vi "Report build (SubVI).vi"(0 "Full/Fails":string(combo)="Full", 1 "Operator":string, 2 "Original ATR Ref":refnum<vi>, 3 "GeneralResult-Pass(T)Fail(F)":bool, 4 "Header Array":string[][](array[string]), 5 "error in (no error)":errorcluster, 6 "report file path":path, 8 "PN":string, 14 "SN":string) -> (19 "error out":errorcluster)   [LabVIEW 2017]
uses:
  <vilib>/Utility/miscctls.llb/LVRowAndColumnUnsignedTypeDef.ctl
  <vilib>/Utility/NIReport.llb/HTML Report Image Alignment.ctl
  <vilib>/Utility/NIReport.llb/Append Image to Report (path wrap).vi
  <vilib>/Utility/NIReport.llb/Append Report Text (str wrap).vi
  <vilib>/Utility/NIReport.llb/Append Text Table to Report (wrap).vi
  <vilib>/Utility/NIReport.llb/NI_report.lvclass
  <vilib>/Utility/NIReport.llb/Word/NI_Word.lvclass
  <vilib>/addons/_office/NI_ReportGenerationToolkit.lvlib
  <vilib>/Utility/NIReport.llb/NI_ReportGenerationCore.lvlib
panel:
  in  "ATR":string[][](table)=[["Comm. & Motor Test", "", "", "", "", "N/A", " ", "", "", "", "", " "], ["RS232 Communication", "", "-", "-", "N/A", "N/A", " ", "", "", "", "", ""], ["Version", "", "-", "-", "N/A", "N/A", "", "", "", "", "", ""], ["Motor Speed", "1000", "-", "-", "N/A", "N/A", "", "", "", "", "", ""], ["Motor Dir.", "1000", "-", "-", "N/A", "N/A", "", "", "", "", "", ""], ["", "", "", "", " ", " ", "", "", "", "", "", ""], ["Motor Thermistor Test", "", "", "", " ", "N/A", "", "", "", "", "", ""], ["Thermistor Disable", "0", "+/-100", "rpm", "N/A", "N/A", "", "", "", "", "", ""], ["Thermistor Enable", "1000", "+/-100", "rpm", "N/A", "N/A", "", "", "", "", "", ""], ["", "", "", "", "", "", "", "", "", "", "", ""], ["Motor Run Test", "", "", "", "", "", "", "", "", "", "", ""], ["Motor Temper. befor Run", "30", "+/-15", "C", "N/A", "N/A", "", "", "", "", "", ""], ["Motor Current after 1 min", "40", "+/-3", "A", "N/A", "N/A", "", "", "", "", "", ""], ["Motor Temper. after 20 min", "45", "+/-15", "C", "N/A", "N/A", "", "", "", "", "", ""], ["Motor Current after 20 min", "40", "+/-3", "A", "N/A", "N/A", "", "", "", "", "", ""], ["", "", "", "", "", "", "", "", "", "", "", ""], ["Visual Inspection Tests", "", "", "", "", "N/A", "", "", "", "", "", ""], ["", "", "", "", "", "", "", "", "", "", "", ""], ["Conductivity Test", "", "", "", "", "N/A", "", "", "", "", "", ""], ["J1 to Chasis", "< 2m", "-", "ohms", "N/A", "N/A", "", "", "", "", "", ""], ["", "", "", "", "", "", "", "", "", "", "", ""], ["Insulation Resistance Test", "", "", "", "", "N/A", "", "", "", "", "", ""], ["J1B", "> 500k", "-", "ohms", "N/A", "N/A", "", "", "", "", "", ""], ["J1E", "> 500k", "-", "ohms", "N/A", "N/A", "", "", "", "", "", ""], ["", "", "", "", "", "", "", "", "", "", "", ""], ["Blower Calibration", "", "", "", "", "N/A", "", "", "", "", "", ""], ["Motor Speed", "8000", "+/-100", "rpm", "N/A", "N/A", "", "", "", "", "", ""], ["Driver Current", "40", "+/-3", "A", "N/A", "N/A", "", "", "", "", "", ""], ["", "", "", "", "", "", "", "", "", "", "", ""], ["Leak Test", "", "", "", "", "N/A", "", "", "", "", "", ""], ["Leak Test", "5", "+/-0.2", "psig", "N/A", "N/A", "", "", "", "", "", ""], ["", "", "", "", "", "", "", "", "", "", "", ""], ["Set Production Parameters", "", "", "", "", "", "", "", "", "", "", ""], ["Unit Serial Number", "#6", "-", "-", "N/A", "N/A", "", "", "", "", "", ""], ["Unit Part Number", "#7", "-", "-", "RD00000", "N/A", "", "", "", "", "", ""]]
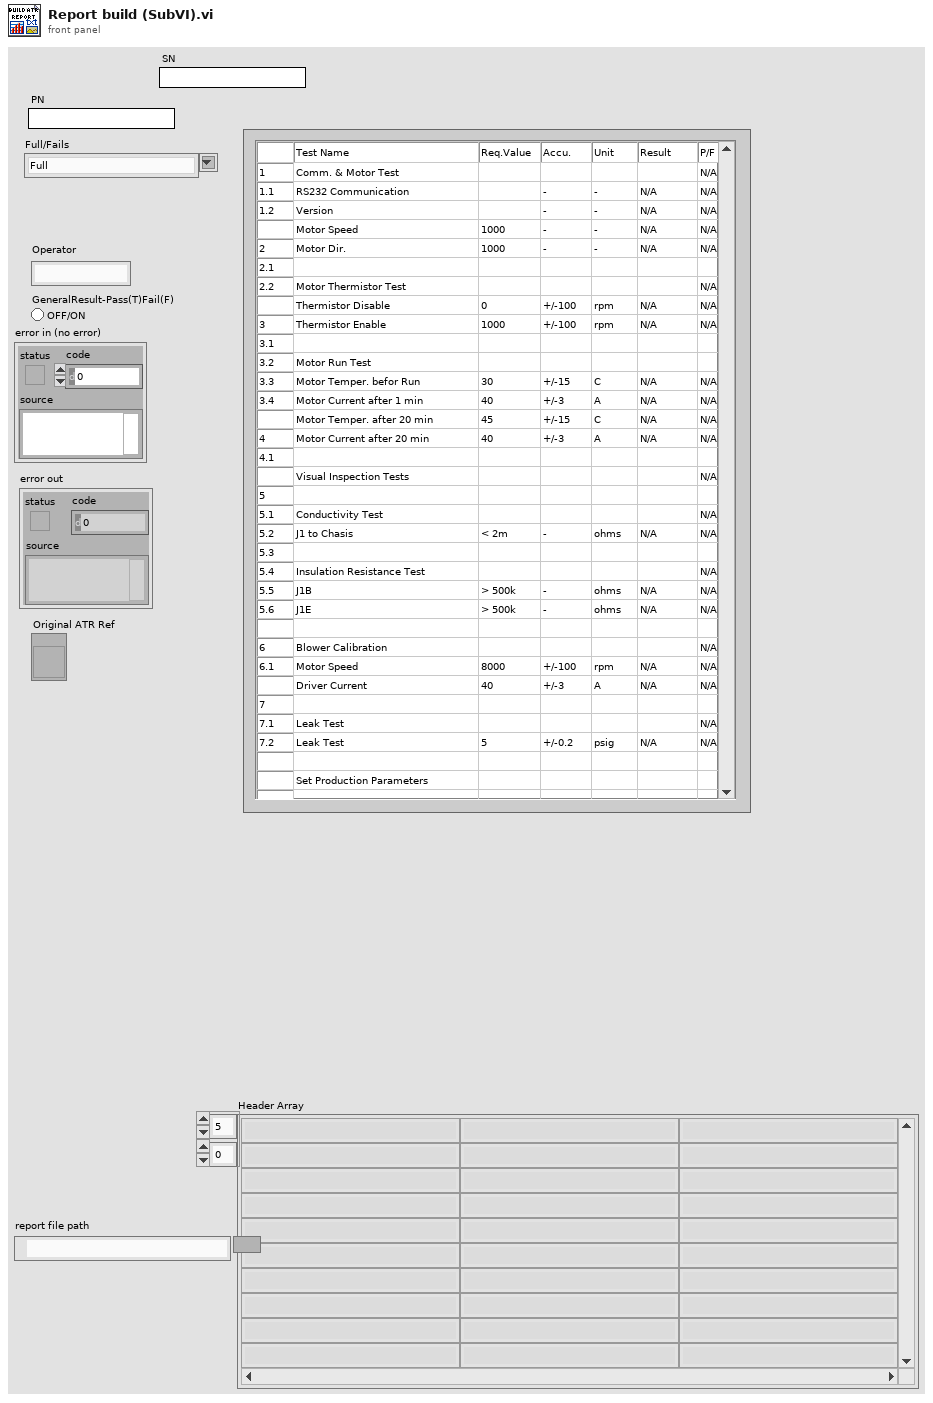
[diagram p1: front panel]
types:
  T1 = cluster{"top":dbl, "left":dbl, "right":dbl, "bottom":dbl}
  T2 = cluster{"alignment":enum16{"Left", "Centered", "Right", "Justify"}, "left":dbl, "right":dbl, "special":enum16{"(none)", "First line", "Hanging"}, "by":dbl, "before":dbl, "after":dbl, "line spacing":enum16{"Single", "1,5 lines", "Double", "At least", "Exactly", "Multiple"}, "at":dbl}
  T3 = enum16{"maximized", "minimized", "normal", "no change"}
  T4 = enum16{"Standard Report", "HTML", "Word", "Excel"}
  T5 = typedef "LVRowAndColumnUnsignedTypeDef.ctl" = cluster{"Row":u32, "Column":u32}
  T6 = typedef "LVFontTypeDef.ctl" = cluster{"Font Name":string, "Size":u16, "Bold":bool, "Italic":bool, "Underline":bool, "Strikeout":bool, "Color":u32}
  T7 = typedef "NI_ReportGenerationCore.lvlib/HTML Report Image Alignment.ctl" = enum16{"(default)", "LEFT", "RIGHT", "TOP", "TEXTTOP", "MIDDLE", "ABSMIDDLE", "BASELINE", "BOTTOM", "ABSBOTTOM"}
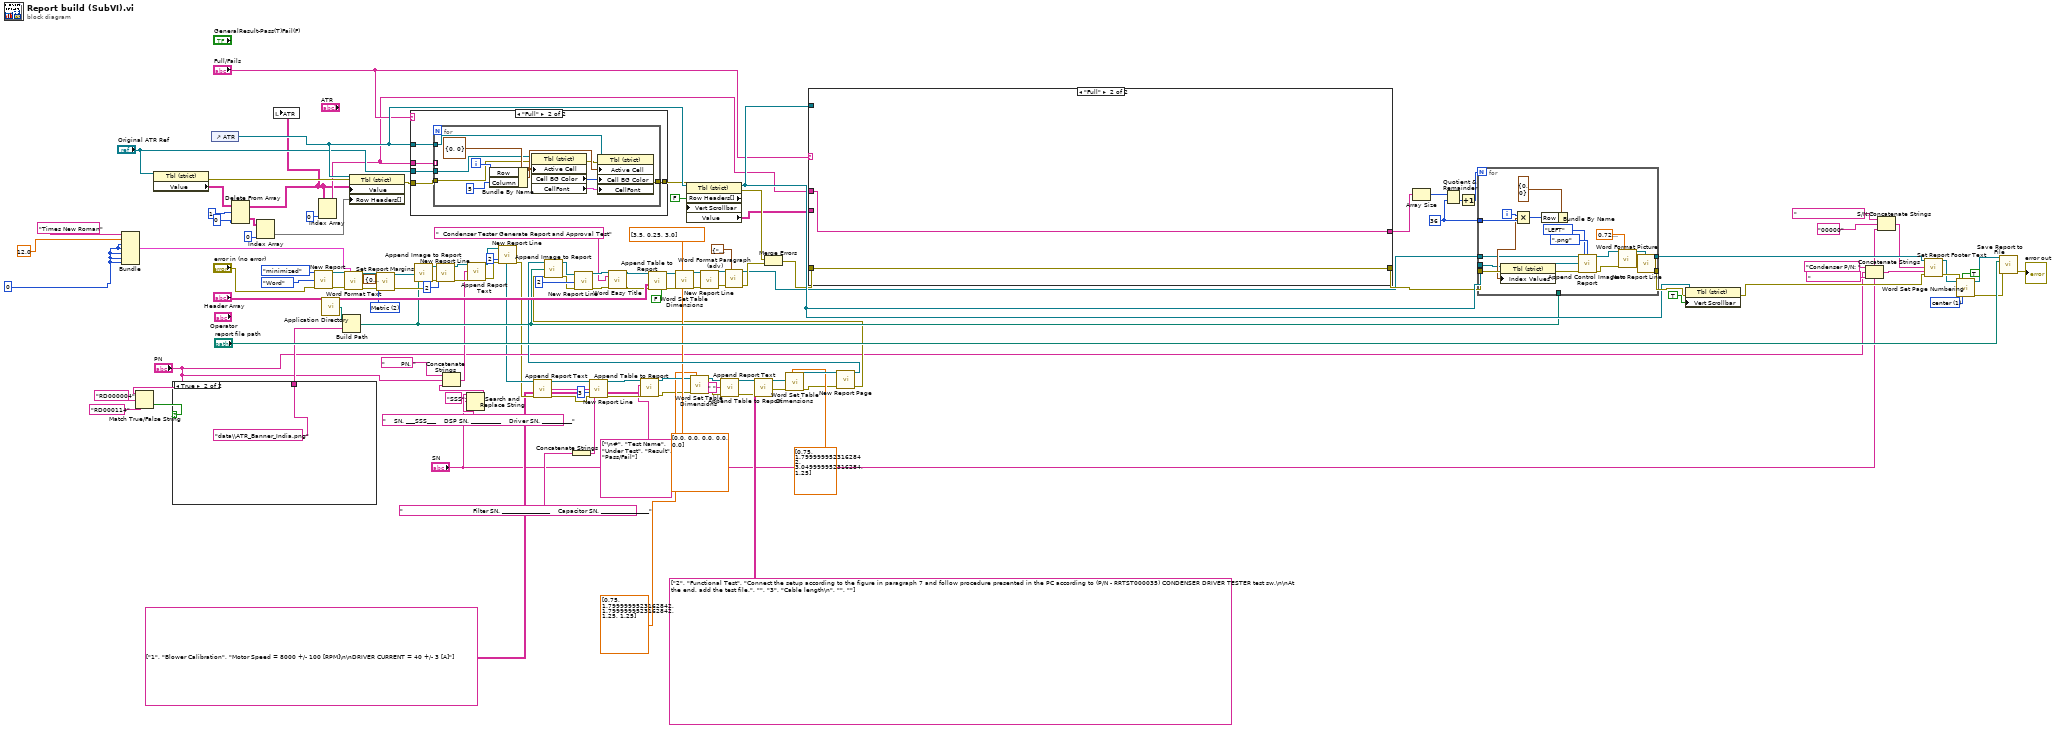
[diagram p0: block diagram]
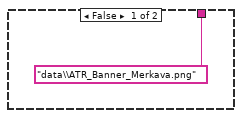
[diagram p2: hidden frame]
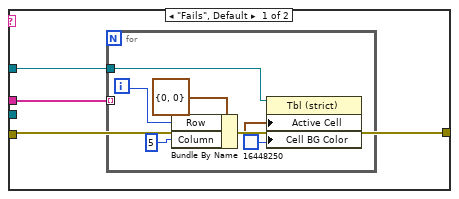
[diagram p3: hidden frame]
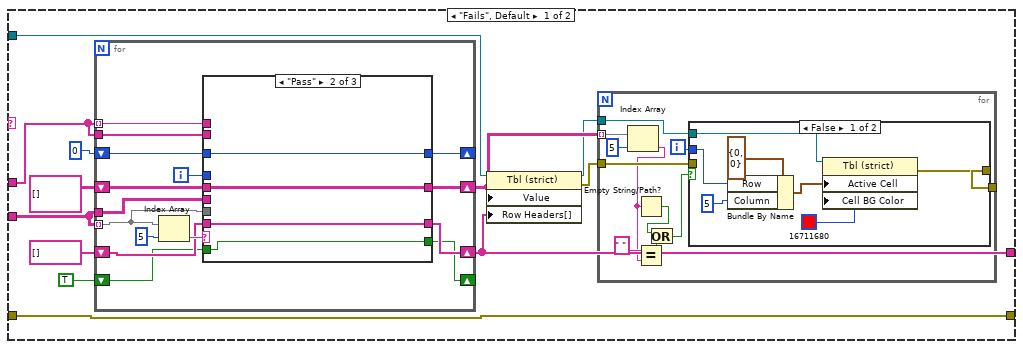
[diagram p4: hidden frame]
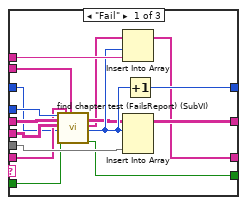
[diagram p6: hidden frame]
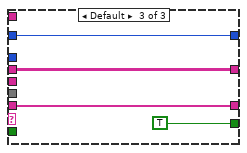
[diagram p7: hidden frame]
diagram:
  w47 = 0
  w78 = u16 1 items=["left", "center", "right"] ("alignment (right)")
  w83 = u16 2 items=["Default", "US", "Metric"] ("measurement system (default)")
  w121 = 36 ("y")
  n1 = Bundle("Times New Roman", 12.0, w47, w47, w47, w47, w47) -> (w50:cluster{string, dbl, i32, i32, i32, i32, i32})  [unwired: 1 in]
  n2 = Match True/False String(2:"RD000114" ("false string"), 3:"RD000004" ("true string"), 4:"PN") -> (0:w70:bool)  [unwired: 1 out]
  n3 = property class="Tbl (strict)"(reference="Original ATR Ref") -> (error out=w95:errorcluster, "Value"=w11:string[][])  [unwired: 1 in, 1 out]
  n4 = case shown="True" w70 {
    tunnel: ["data\\ATR_Banner_Merkava.png" ("name or relative path") "data\\ATR_Banner_India.png" ("name or relative path")] -> w69
    frame False {
    }
    frame True {
    }
  }
  n5 = control-ref of="ATR"() -> (w114:refnum<vi>)
  n6 = Delete From Array(array=w11, length=1, index (col)=0 ("disabled index (col)")) -> (deleted portion=w8:string[][], array with subset deleted=w5:string[][])  [unwired: 1 in]
  n7 = Index Array(array=w8, index (col)=0 ("disabled index (col)")) -> (element=w6:string[])  [unwired: 1 in]
  n8 = local write "ATR"(w5) -> ()
  n9 = call <vilib>:"New Report.vi"("window state (normal)"=T3."minimized", "report type"=T4."Word", "error in (no error)"="error in (no error)") -> ("report out"=w54:refnum<class "NI_report.lvclass">, "error out"=w51:errorcluster)  [unwired: 11 in]
  n10 = Index Array(array=w5, index (col)=0 ("disabled index (col)")) -> (element=w85:string[])  [unwired: 1 in]
  n11 = call <vilib>:"Application Directory.vi"() -> ("Application Directory"=w82:path)
  n12 = Build Path(base path=w82, name or relative path=w69) -> (appended path=w65:path)
  n13 = call <vilib>:"Word Format Text.vi"("report in"=w54, "font"=w50, "error in (no error)"=w51) -> ("report out"=w53:refnum<class "NI_report.lvclass">, "error out"=w52:errorcluster)  [unwired: 11 in]
  n14 = property class="Tbl (strict)"(reference=w114, error in=w95, "Value"=w5, "Row Headers[]"=w6) -> (error out=w112:errorcluster)  [unwired: 1 out]
  n15 = call-dynamic "Set Report Margins.vi"("report in"=w53, "margins (1.00)"=T1 {"top"=0.1, "left"=2.5, "right"=1.0, "bottom"=0.75}, "measurement system (default)"=w83, "error in (no error)"=w52) -> ("report out"=w81:refnum<class "NI_report.lvclass">, "error out"=w80:errorcluster)  [unwired: 9 in, 1 out]
  n16 = case shown="\"Full\"" "Full/Fails" {
    tunnel: w114 -> [w128 w141]
    tunnel: "Original ATR Ref" -> [_ w140]
    tunnel: [w130 w139] -> w113
    tunnel: w112 -> [w130 w138]
    tunnel: w85 -> [w129 w137]
    frame "Fails", Default {
      n17 = for {
        tunnel: w129 -> [_] mode=indexing
        tunnel: w128 -> [w131]
        i -> [w136]
        n18 = Bundle By Name(cluster=T5 {"Row"=0, "Column"=0} ("Index Values"), "Row"=w136, "Column"=u32 5) -> (w134:T5)
        n19 = property class="Tbl (strict)"(reference=w131, "Active Cell"=w134, "Cell BG Color"=u32 16448250) -> ()  [unwired: 1 in, 2 out]
      }
    }
    frame "Full" {
      n20 = for {
        tunnel: w141 -> [w146]
        tunnel: w140 -> [w145]
        tunnel: [w144] -> w139
        tunnel: w138 -> [w142]
        tunnel: w137 -> [_] mode=indexing
        i -> [w147]
        n21 = Bundle By Name(cluster=T5 {"Row"=0, "Column"=0} ("Index Values"), "Row"=w147, "Column"=u32 5) -> (w149:T5)
        n22 = property class="Tbl (strict)"(reference=w145, error in=w142, "Active Cell"=w149) -> (error out=w143:errorcluster, "Cell BG Color"=w152:u32, "CellFont"=w151:T6)  [unwired: 1 out]
        n23 = property class="Tbl (strict)"(reference=w146, error in=w143, "Active Cell"=w149, "Cell BG Color"=w152, "CellFont"=w151) -> (error out=w144:errorcluster)  [unwired: 1 out]
      }
    }
  }
  n24 = call-poly <vilib>:"Append Image to Report.vi"("report in"=w81, "path or URL of image"=w65, "error in (no error)"=w80) -> ("report out"=w77:refnum<class "NI_report.lvclass">, "error out"=w45:errorcluster)  [unwired: 9 in, 2 out]
  n25 = call-dynamic "New Report Line.vi"("report in"=w77, "number of lines (1)"=2) -> ("report out"=w36:refnum<class "NI_report.lvclass">)  [unwired: 12 in, 1 out]
  n26 = Search and Replace String(input string="    SN. ___SSS___    DSP SN. __________    Driver SN. __________" ("string"), search string="SSS", replace string="SN") -> (result string=w4:string)  [unwired: 5 in, 3 out]
  n27 = Concatenate Strings("        PN. " ("string"), "PN", w4) -> (w42:string)
  n28 = call-poly <vilib>:"Append Report Text.vi"("report in"=w36, "text"=w42, "error in (no error)"=w45) -> ("report out"=w46:refnum<class "NI_report.lvclass">, "error out"=w35:errorcluster)  [unwired: 9 in, 2 out]
  n29 = call-dynamic "New Report Line.vi"("report in"=w46, "number of lines (1)"=2, "error in (no error)"=w35) -> ("report out"=w39:refnum<class "NI_report.lvclass">, "error out"=w34:errorcluster)  [unwired: 11 in]
  n30 = Concatenate Strings("                                   Filter SN. ________________    Capacitor SN. ________________" ("string")) -> (w33:string)
  n31 = call-poly <vilib>:"Append Report Text.vi"("report in"=w39, "text"=w33, "error in (no error)"=w34) -> ("report out"=w38:refnum<class "NI_report.lvclass">, "error out"=w27:errorcluster)  [unwired: 9 in, 2 out]
  n32 = call-dynamic "New Report Line.vi"("report in"=w38, "number of lines (1)"=3, "error in (no error)"=w27) -> ("report out"=w30:refnum<class "NI_report.lvclass">, "error out"=w26:errorcluster)  [unwired: 11 in]
  n33 = call-poly <vilib>:"Append Table to Report.vi"("report in"=w30, "column headers"=string[] ["\n#", "Test Name", "Under Test", "Result", "Pass/Fail"], "text data"=string[][] [["1", "Blower Calibration", "Motor Speed = 8000 +/- 100 [RPM]\n\nDRIVER CURRENT = 40 +/- 3 [A]"]], "error in (no error)"=w26) -> ("report out"=w28:refnum<class "NI_report.lvclass">, "error out"=w22:errorcluster)  [unwired: 8 in, 2 out]
  n34 = property class="Tbl (strict)" props=["Row Headers[]", "Vert Scrollbar", "Value"](reference=w114, error in=w113, "Vert Scrollbar"=FALSE ("Visible Items:Vertical Scrollbar Visible")) -> (reference out=w116:refnum<vi>, error out=w98:errorcluster, "Value"=w68:string[][])  [unwired: 1 out]
  n35 = call <vilib>:"Word Set Table Dimensions.vi"("report in"=w28, "table column widths"=sgl[] [0.75, 1.8, 1.8, 1.25, 1.25], "error in (no error)"=w22) -> ("report out"=w15:refnum<class "NI_report.lvclass">, "error out"=w14:errorcluster)  [unwired: 11 in]
  n36 = call-poly <vilib>:"Append Report Text.vi"("report in"=w15, "text"=" ") -> ("report out"=w13:refnum<class "NI_report.lvclass">)  [unwired: 10 in, 3 out]
  n37 = call-poly <vilib>:"Append Table to Report.vi"("report in"=w13, "text data"=string[][] [["2", "Functional Test", "Connect the setup according to the figure in paragraph 7 and follow procedure presented in the PC according to (P/N - RRTST000035) CONDENSER DRIVER TESTER test sw.\n\nAt the end, add the test file.", ""], ["3", "Cable length\n", "", ""]], "error in (no error)"=w14) -> ("report out"=w21:refnum<class "NI_report.lvclass">, "error out"=w17:errorcluster)  [unwired: 9 in, 2 out]
  n38 = call <vilib>:"Word Set Table Dimensions.vi"("report in"=w21, "table column widths"=sgl[] [0.75, 1.8, 3.05, 1.25], "error in (no error)"=w17) -> ("report out"=w19:refnum<class "NI_report.lvclass">, "error out"=w16:errorcluster)  [unwired: 11 in]
  n39 = call-dynamic "New Report Page.vi"("report in"=w19, "error in (no error)"=w16) -> ("report out"=w67:refnum<class "NI_report.lvclass">, "error out"=w44:errorcluster)  [unwired: 12 in]
  n40 = call-poly <vilib>:"Append Image to Report.vi"("report in"=w67, "path or URL of image"=w65, "error in (no error)"=w44) -> ("report out"=w66:refnum<class "NI_report.lvclass">, "error out"=w43:errorcluster)  [unwired: 9 in, 2 out]
  n41 = call-dynamic "New Report Line.vi"("report in"=w66, "number of lines (1)"=2, "error in (no error)"=w43) -> ("report out"=w91:refnum<class "NI_report.lvclass">, "error out"=w90:errorcluster)  [unwired: 11 in]
  n42 = call <vilib>:"Word Easy Title.vi"("report in"=w91, "title"="  Condenser Tester Generate Report and Approval Test" ("text"), "error in (no error)"=w90) -> ("report out"=w88:refnum<class "NI_report.lvclass">, "error out"=w89:errorcluster)  [unwired: 10 in, 1 out]
  n43 = call-poly <vilib>:"Append Table to Report.vi"("report in"=w88, "text data"="Header Array", "error in (no error)"=w89, "show grid lines (YES)"=FALSE) -> ("report out"=w107:refnum<class "NI_report.lvclass">, "error out"=w106:errorcluster)  [unwired: 8 in, 2 out]
  n44 = call <vilib>:"Word Set Table Dimensions.vi"("report in"=w107, "table column widths"=sgl[] [3.5, 0.25, 3.0], "error in (no error)"=w106, "table row heights"=sgl[] [0.0, 0.0, 0.0, 0.0, 0.0]) -> ("report out"=w101:refnum<class "NI_report.lvclass">, "error out"=w100:errorcluster)  [unwired: 10 in]
  n45 = call-dynamic "New Report Line.vi"("report in"=w101) -> ("report out"=w55:refnum<class "NI_report.lvclass">)  [unwired: 13 in, 1 out]
  n46 = call <vilib>:"Word Format Paragraph (adv).vi"("report in"=w55, "indent and spacing"=T2 {"alignment"=enum."Left", "left"=0.0, "right"=0.0, "special"=enum."(none)", "by"=0.0, "before"=0.0, "after"=0.0, "line spacing"=enum."Single", "at"=0.0}, "error in (no error)"=w100) -> ("report out"=w64:refnum<class "NI_report.lvclass">, "error out"=w97:errorcluster)  [unwired: 11 in]
  n47 = Merge Errors(w98, w97) -> (w96:errorcluster)
  n48 = case shown="\"Full\"" "Full/Fails" {
    tunnel: w96 -> [w164 w223]
    tunnel: w85 -> [w159 w224]
    tunnel: [w164 w223] -> w115
    tunnel: w68 -> [w160 _]
    tunnel: [w156 w224] -> w119
    tunnel: w116 -> [w157 _]
    frame "Fails", Default {
      n49 = for {
        tunnel: w160 -> [w192] mode=indexing
        shift-right: [w194] -> w155
        shift-left: string[][] [] -> [w196]
        shift-right: [w193] -> _
        shift-left: 0 -> [w195]
        tunnel: w159 -> [w190] mode=indexing
        shift-right: [w189] -> w156
        shift-left: string[] [] -> [w191]
        tunnel: w160 -> [w187]
        tunnel: w159 -> [w186]
        shift-right: [w184] -> _
        shift-left: TRUE -> [w185]
        i -> [w188]
        n50 = Index Array(array=w192, index=5) -> (element=w197:string)
        n51 = case shown="\"Pass\"" w197 {
          tunnel: w196 -> [w208 w217 w221]
          tunnel: w195 -> [w205 w218 w222]
          tunnel: [w214 w217 w221] -> w194
          tunnel: [w213 w218 w222] -> w193
          tunnel: w192 -> [w212 _ _]
          tunnel: w191 -> [w207 w216 w220]
          tunnel: w190 -> [w206 _ _]
          tunnel: [w211 w216 w220] -> w189
          tunnel: w188 -> [w209 _ _]
          tunnel: w187 -> [w210 _ _]
          tunnel: w186 -> [w201 _ _]
          tunnel: w185 -> [w200 w215 _]
          tunnel: [w199 w215 TRUE ("ToExecute? Out")] -> w184
          frame "Fail" {
            n52 = call "find chapter test (FailsReport) (SubVI).vi"("ForLoopIndex"=w209, "Fails ATR IN"=w208, "Full ATR"=w210, "FailsATR Index IN"=w205, "ToExecute?"=w200, "Fails ATR RowHeader IN"=w207, "Full ATR RowHeader"=w201) -> ("Fails ATR OUT"=w203:string[][], "Fails ATR RowHeader OUT"=w202:string[], "FailsATR Index OUT"=w204:i32, "ToExecute? Out"=w199:bool)  [unwired: 9 in]
            n53 = Insert Into Array(array=w202, index=w204, new element=w206) -> (w211:string[])
            n54 = Insert Into Array(array=w203, index (row)=w204, new element=w212) -> (w214:string[][])  [unwired: 1 in]
            n55 = Increment(x=w204) -> (x+1=w213:i32)
          }
          frame "Pass" {
          }
          frame Default {
          }
        }
      }
      n56 = property class="Tbl (strict)"(reference=w157, "Value"=w155, "Row Headers[]"=w156) -> (reference out=w153:refnum<vi>, error out=w154:errorcluster)  [unwired: 1 in]
      n57 = for {
        tunnel: [w174] -> _
        tunnel: w155 -> [w173] mode=indexing
        tunnel: w154 -> [w171]
        tunnel: w153 -> [w170]
        i -> [w175]
        n58 = Index Array(array=w173, index=5) -> (element=w167:string)
        n59 = Empty String/Path?(string/path=w167) -> (empty?=w169:bool)
        n60 = Equal?(x=" ", y=w167) -> (x = y?=w166:bool)
        n61 = Or(x=w169, y=w166) -> (x .or. y?=w165:bool)
        n62 = case shown="False" w165 {
          tunnel: w175 -> [w179 _]
          tunnel: [w178 w183] -> w174
          tunnel: w171 -> [_ w183]
          tunnel: w170 -> [w176 _]
          frame False {
            n63 = Bundle By Name(cluster=T5 {"Row"=0, "Column"=0} ("Index Values"), "Row"=w179, "Column"=u32 5) -> (w181:T5)
            n64 = property class="Tbl (strict)"(reference=w176, "Active Cell"=w181, "Cell BG Color"=u32 16711680) -> (error out=w178:errorcluster)  [unwired: 1 in, 1 out]
          }
          frame True {
          }
        }
      }
    }
    frame "Full" {
    }
  }
  n65 = Array Size(array=w119) -> (size(s)=w122:i32)
  n66 = Quotient & Remainder(x=w122, y=w121) -> (floor(x/y)=w123:i32)  [unwired: 1 out]
  n67 = Increment(x=w123) -> (x+1=w124:i32)
  n68 = for {
    N: w124 -> [_]
    tunnel: w121 -> [w239]
    tunnel: w64 -> [w232]
    tunnel: w115 -> [w237]
    tunnel: [w228] -> w117
    tunnel: w116 -> [w234]
    tunnel: [w226] -> w110
    tunnel: w65 -> [_]
    i -> [w240]
    n69 = Multiply(x=w240, y=w239) -> (x*y=w241:i32)
    n70 = Bundle By Name(cluster=T5 {"Row"=0, "Column"=0} ("Index Values"), "Row"=w241) -> (w236:T5)
    n71 = property class="Tbl (strict)"(reference=w234, error in=w237, "Index Values"=w236) -> (reference out=w235:refnum<vi>, error out=w233:errorcluster)
    n72 = call-dynamic "Append Control Image to Report.vi"("report in"=w232, "alignment (default)"=HTML_Report_Image_Alignment."LEFT", "image file type (.jpg)"=enum16{".jpg", ".png"}.".png" ("image file type(.jpg)"), "ctrl reference"=w235, "error in (no error)"=w233) -> ("report out"=w231:refnum<class "NI_report.lvclass">, "error out"=w229:errorcluster)  [unwired: 7 in, 2 out]
    n73 = call <vilib>:"Word Format Picture.vi"("report in"=w231, "scale factor (1)"=sgl 0.72, "error in (no error)"=w229) -> ("report out"=w230:refnum<class "NI_report.lvclass">, "error out"=w228:errorcluster)  [unwired: 11 in]
    n74 = call-dynamic "New Report Line.vi"("report in"=w230) -> ("report out"=w226:refnum<class "NI_report.lvclass">)  [unwired: 13 in, 1 out]
  }
  n75 = property class="Tbl (strict)"(reference=w116, error in=w117, "Vert Scrollbar"=TRUE ("Visible Items:Vertical Scrollbar Visible")) -> (error out=w109:errorcluster)  [unwired: 1 out]
  n76 = Concatenate Strings("Condenser P/N: " ("left footer text"), "PN", "                           " ("string")) -> (w58:string)
  n77 = Concatenate Strings("                              S/N: " ("string"), "00000" ("string"), "SN") -> (w56:string)
  n78 = call-dynamic "Set Report Footer Text.vi"("report in"=w110, "center footer text"=w56, "right footer text"=w58, "error in (no error)"=w109) -> ("report out"=w75:refnum<class "NI_report.lvclass">, "error out"=w76:errorcluster)  [unwired: 10 in]
  n79 = call <vilib>:"Word Set Page Numbering.vi"("report in"=w75, "include page x of n"=TRUE, "alignment (right)"=w78, "error in (no error)"=w76) -> ("report out"=w73:refnum<class "NI_report.lvclass">, "error out"=w74:errorcluster)  [unwired: 10 in]
  n80 = call-dynamic "Save Report to File.vi"("report in"=w73, "report file path"="report file path", "error in (no error)"=w74) -> ("error out"=→"error out":errorcluster)  [unwired: 11 in, 1 out]
